vi "Ophir Measure.vi"(4 "error in (no error)":errorcluster, 5 "Power Method ?(0)":i32, 6 "Measure Choice (0:Power)":u16(ring) items=["Power", "Energy", "Frequency"], 7 "Visa Session":refnum<visa-resource-name>) -> (0 "error out":errorcluster, 1 "Value String":string, 2 "Value Number":dbl format="%.3e", 3 "dup Visa Session":refnum<visa-resource-name>)   [LabVIEW 2017]
doc: "Measure.vi executes measurement specified in Measure Choice\nVersion 1.00\nLast Updated 16 May 2002\n\nInputs:\nVISA Session.\nMeasure Choice :\nMenu to select what to measure.\n0 for Power\n1 for Energy\n2 for Frequency\ndefault 0:Power\nPower Method: number of method for Power Measurement\n 0 for none method\n 1 for ThermoPile + PhotoDiode head\n 2 for PyroElectric + NanoJoule-Meter head\ndefault:0\nErrorIn\n\nOutputs:\ndup Visa Session \nValue Number is the measurement value\nValue String is the measurement string\n\nNote:\nIn case of Overrange Measure The string contains *OVER\nErrorOut:"
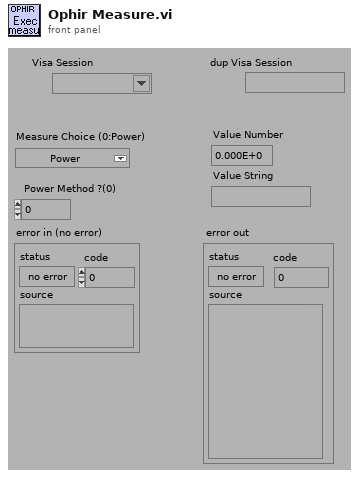
[diagram p1: front panel]
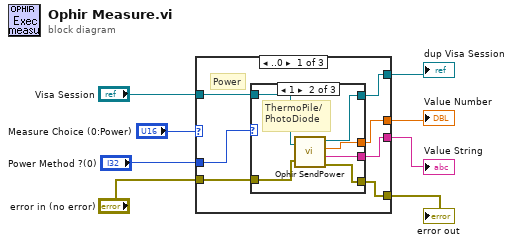
[diagram p0: block diagram]
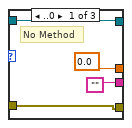
[diagram p2: hidden frame]
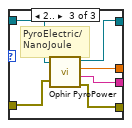
[diagram p3: hidden frame]
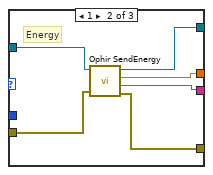
[diagram p4: hidden frame]
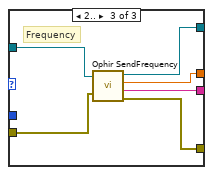
[diagram p5: hidden frame]
diagram:
  n1 = case shown="..0" "Measure Choice (0:Power)" {
    tunnel: "Visa Session" -> [w15 w37 w43]
    tunnel: [w14 w36 w42] -> w6
    tunnel: "error in (no error)" -> [w13 w35 w41]
    tunnel: [w12 w34 w40] -> w4
    tunnel: [w10 w32 w39] -> w3
    tunnel: [w11 w33 w38] -> w2
    tunnel: "Power Method ?(0)" -> [w9 _ _]
    frame ..0 {
      # "Power"
      n2 = case shown="1" w9 {
        tunnel: w15 -> [w19 w25 w31]
        tunnel: [w19 w24 w30] -> w14
        tunnel: w13 -> [w18 w23 w26]
        tunnel: [w18 w22 w27] -> w12
        tunnel: [0.0 w21 w29] -> w11
        tunnel: ["" w20 w28] -> w10
        frame ..0 {
          # "No Method"
        }
        frame 1 {
          # "ThermoPile/\nPhotoDiode"
          n3 = call "Ophir SendPower.vi"("Visa Session"=w25, "error in (no error)"=w23) -> ("dup Visa Session"=w24:refnum<visa-resource-name>, "Value Number"=w21:dbl, "Value String"=w20:string, "error out"=w22:errorcluster)
        }
        frame 2.. {
          # "PyroElectric/\nNanoJoule"
          n4 = call "Ophir PyroPower.vi"("Visa Session"=w31, "error in (no error)"=w26) -> ("dup Visa Session"=w30:refnum<visa-resource-name>, "Value Number"=w29:dbl, "Value String"=w28:string, "error out"=w27:errorcluster)
        }
      }
    }
    frame 1 {
      # "Energy"
      n5 = call "Ophir SendEnergy.vi"("Visa Session"=w37, "error in (no error)"=w35) -> ("dup Visa Session"=w36:refnum<visa-resource-name>, "Value Number"=w33:dbl, "Value String"=w32:string, "error out"=w34:errorcluster)  [unwired: 1 out]
    }
    frame 2.. {
      # "Frequency"
      n6 = call "Ophir SendFrequency.vi"("Visa Session"=w43, "error in (no error)"=w41) -> ("dup Visa Session"=w42:refnum<visa-resource-name>, "Value Number"=w38:dbl, "Value String"=w39:string, "error out"=w40:errorcluster)
    }
  }
  "error out" <- w4
  "dup Visa Session" <- w6
  "Value String" <- w3
  "Value Number" <- w2
